vi "Generate.vi"(9 "Reset":bool, 10 "Gen Params":T2, 11 "Timing Params":T1) -> (2 "signal out":waveform(dbl))   [LabVIEW 2020, in "WaveGen.lvlib"]
uses:
  WaveGen.lvlib
  <vilib>/measure/NI_MABase.lvlib
  Shape.ctl
  Signal Params.ctl
  Timing Params.ctl
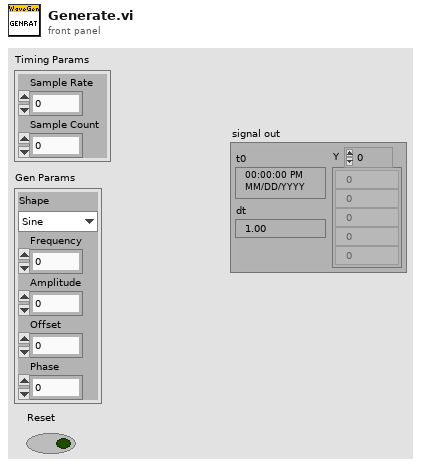
[diagram p1: front panel]
types:
  T1 = typedef "WaveGen.lvlib/Timing Params.ctl" = cluster{"Sample Rate":dbl, "Sample Count":dbl}
  T2 = typedef "WaveGen.lvlib/Signal Params.ctl" = cluster{"Shape":T3, "Frequency":dbl, "Amplitude":dbl, "Offset":dbl, "Phase":dbl}
  T3 = typedef "WaveGen.lvlib/Shape.ctl" = enum16{"Sine", "Square", "Triangle", "Saw"}
  T4 = enum16{"Sine Wave", "Triangle Wave", "Square Wave", "Sawtooth Wave"}
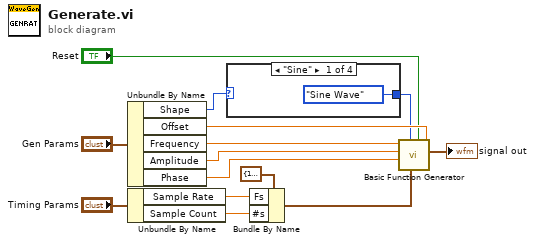
[diagram p0: block diagram]
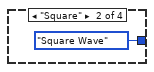
[diagram p2: hidden frame]
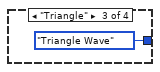
[diagram p3: hidden frame]
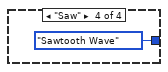
[diagram p4: hidden frame]
diagram:
  n1 = Unbundle By Name("Gen Params") -> ("Shape"=w13:T3, "Offset"=w10:dbl, "Frequency"=w11:dbl, "Amplitude"=w7:dbl, "Phase"=w6:dbl)
  n2 = Unbundle By Name("Timing Params") -> ("Sample Rate"=w3:dbl, "Sample Count"=w2:dbl)
  n3 = case shown="\"Sine\"" w13 {
    tunnel: [T4."Sine Wave" ("signal type") T4."Square Wave" ("signal type") T4."Triangle Wave" ("signal type") T4."Sawtooth Wave" ("signal type")] -> w8
    frame "Sine" {
    }
    frame "Square" {
    }
    frame "Triangle" {
    }
    frame "Saw" {
    }
  }
  n4 = Bundle By Name(cluster=cluster{"Fs":dbl, "#s":dbl} {"Fs"=1000.0, "#s"=1000.0} ("sampling info"), "Fs"=w3, "#s"=w2) -> (w4:cluster{"Fs":dbl, "#s":dbl})
  n5 = call <vilib>:"Basic Function Generator.vi"("offset"=w10, "reset signal"="Reset", "sampling info"=w4, "signal type"=w8, "phase"=w6, "amplitude"=w7, "frequency"=w11) -> ("signal out"=→"signal out":waveform(dbl))  [unwired: 2 in, 2 out]
